vi "Wait.vi"(9 "Target Time (s)":dbl, 11 "First Time?":bool) -> (3 "Completed":bool)   [LabVIEW 2016]
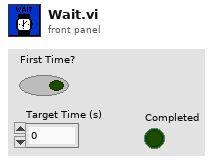
[diagram p1: front panel]
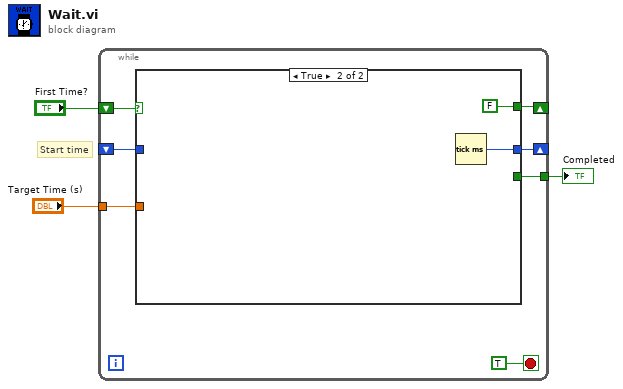
[diagram p0: block diagram]
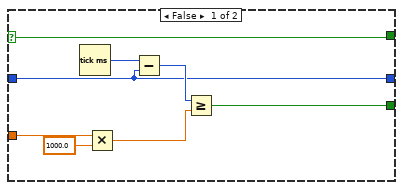
[diagram p2: hidden frame]
diagram:
  # "Start time"
  n1 = while {
    shift-right: [w8] -> _
    shift-left: "First Time?" -> [w9]
    shift-right: [w7] -> _
    shift-left: _ -> [w6]
    tunnel: "Target Time (s)" -> [w5]
    tunnel: [w4] -> w1
    stop <- TRUE stop-if-true
    n2 = case shown="True" w9 {
      selector: w9 -> [w18 _]
      tunnel: [w18 FALSE] -> w8
      tunnel: [w15 w19] -> w7
      tunnel: w6 -> [w15 _]
      tunnel: w5 -> [w14 _]
      tunnel: [w11 _] -> w4
      frame False {
        n3 = Tick Count (ms)() -> (millisecond timer value=w17:u32)
        n4 = Multiply(x=w14, y=1000.0) -> (x*y=w12:dbl)
        n5 = Subtract(x=w17, y=w15) -> (x-y=w16:u32)
        n6 = Greater Or Equal?(x=w16, y=w12) -> (x >= y?=w11:bool)
      }
      frame True {
        n7 = Tick Count (ms)() -> (millisecond timer value=w19:u32)
      }
    }
  }
  "Completed" <- w1
